vi "ICNC Read Parameter.vi"(8 "error in (no error)":errorcluster caption="entrée d'erreur (pas d'erreur)", 10 "ParameterValue":i32, 11 "ParameterID":u32) -> (0 "error out":errorcluster caption="sortie d'erreur", 2 "ParameterValue out":i32, 3 "function return":u32)   [LabVIEW 2012, in "ICNC2.lvlib"]
doc: "DWORD ICNC_ReadParameter( DWORD ParameterID,\n INT *ParameterValue);"
uses:
  <userlib>/ICNC/ICNC2.lvlib
  <userlib>/ICNC/ICNC2.dll
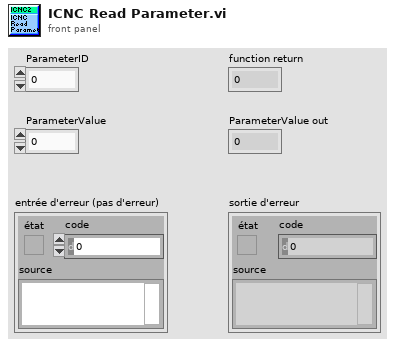
[diagram p1: front panel]
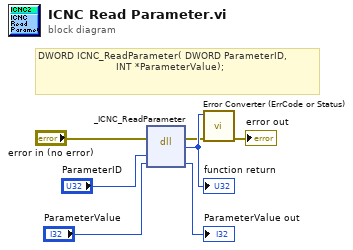
[diagram p0: block diagram]
diagram:
  # "DWORD ICNC_ReadParameter( DWORD ParameterID,\n                          INT *ParameterValue);"
  n1 = dll-call lib="C:/Program Files (x86)/National Instruments/LabVIEW 2012/user.lib/ICNC/ICNC2.*" fn="_ICNC_ReadParameter"(error in="error in (no error)", "ParameterID"="ParameterID", "ParameterValue"="ParameterValue") -> (error out=w2:errorcluster, w7:u32, "ParameterValue"=→"ParameterValue out":i32)  [unwired: 3 in, 1 out]
  "function return" <- w7
  n2 = call <userlib>:"Error Converter (ErrCode or Status).vi"("error in (no error)"=w2, "error code"=w7) -> ("error out"=→"error out":errorcluster)  [unwired: 9 in]
